vi "Command Settings.vi"() -> (5 "Command Settings":T1[](array[typedef])=[{"Enum"=enum."Start", "U8"=0, " Payload"=TRUE}, {"Enum"=enum."Pause", "U8"=0, " Payload"=FALSE}, {"Enum"=enum."Pause", "U8"=0, " Payload"=TRUE}, {"Enum"=enum."Stop", "U8"=0, " Payload"=TRUE}, {"Enum"=enum."RefreshStats", "U8"=0, " Payload"=TRUE}, {"Enum"=enum."UpdateConfig", "U8"=0, " Payload"=FALSE}, {"Enum"=enum."RefreshStats", "U8"=0, " Payload"=TRUE}, {"Enum"=enum."UpdateConfig", "U8"=0, " Payload"=FALSE}, {"Enum"=enum."Start", "U8"=0, " Payload"=FALSE}, {"Enum"=enum."UpdateConfig", "U8"=0, " Payload"=FALSE}])   [LabVIEW 2021, in "CIFCoreOOB_Rx.lvclass"]
uses:
  CIFCoreOOB_Rx.lvclass
  Typedef/Command Setting Control.ctl
  Typedef/OOB Core Commands.ctl
  CIFCoreOOB_Rx.lvclass/CIFCoreOOB_Rx.ctl
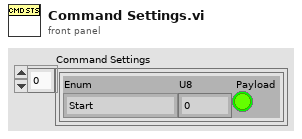
[diagram p1: front panel]
types:
  T1 = typedef "CIFCoreOOB_Rx.lvclass/Command Setting Control.ctl" = cluster{"Enum":T2, "U8":u8, " Payload":bool}
  T2 = typedef "CIFCoreOOB_Rx.lvclass/OOB Core Commands.ctl" = enum8{"Start", "Pause", "Stop", "RefreshStats", "UpdateConfig", "Connect Channel"}
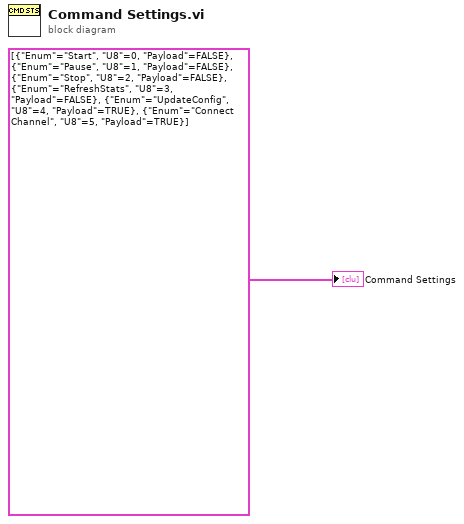
[diagram p0: block diagram]
diagram:
  "Command Settings" <- cluster{"Enum":T2, "U8":u8, "Payload":bool}[] [{"Enum"=enum."Start", "U8"=0, "Payload"=FALSE}, {"Enum"=enum."Pause", "U8"=1, "Payload"=FALSE}, {"Enum"=enum."Stop", "U8"=2, "Payload"=FALSE}, {"Enum"=enum."RefreshStats", "U8"=3, "Payload"=FALSE}, {"Enum"=enum."UpdateConfig", "U8"=4, "Payload"=TRUE}, {"Enum"=enum."Connect Channel", "U8"=5, "Payload"=TRUE}]
